vi "Global N-Back Setting.vi"() -> ()   [LabVIEW 2020]
panel:
  out "N-Back":u8
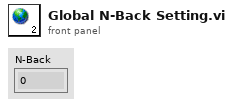
[diagram p1: front panel]
diagram:
